vi "Calc Total Time SubVi.vi"(1 "Vel":dbl, 2 "rep":u32, 3 "Y length":dbl, 4 "X length":dbl) -> (0 "Total Time":dbl)   [LabVIEW 2017]
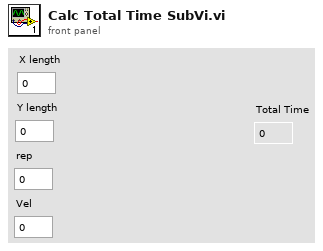
[diagram p1: front panel]
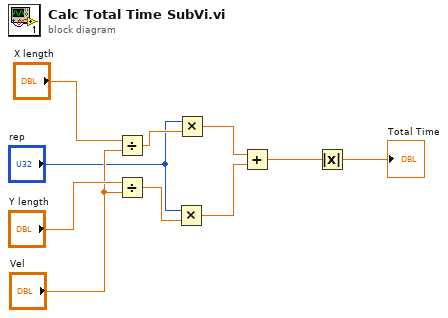
[diagram p0: block diagram]
diagram:
  n1 = Divide(x="X length", y="Vel") -> (x/y=w9:dbl)
  n2 = Divide(x="Y length", y="Vel") -> (x/y=w6:dbl)
  n3 = Multiply(x="rep", y=w6) -> (x*y=w3:dbl)
  n4 = Multiply(x="rep", y=w9) -> (x*y=w4:dbl)
  n5 = Add(x=w4, y=w3) -> (x+y=w2:dbl)
  n6 = Absolute Value(x=w2) -> (abs(x)=→"Total Time":dbl)
